vi "SelectMonitor.vi"(8 "Error In":errorcluster, 9 "Center?":bool, 10 "Monitor (0=primary)":u16, 11 "VI Path":path) -> (0 "Error out":errorcluster)   [LabVIEW 2012, in "LV-Utilities.lvlib"]
uses:
  LV-Utilities.lvlib
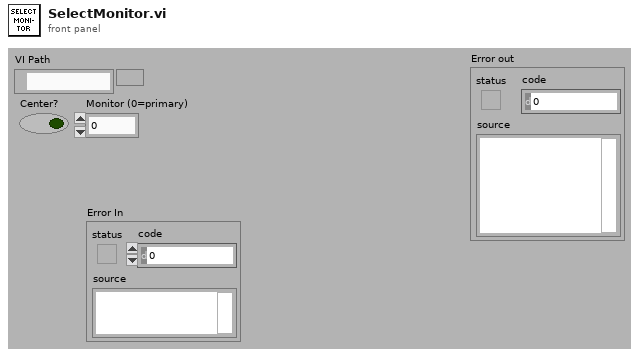
[diagram p1: front panel]
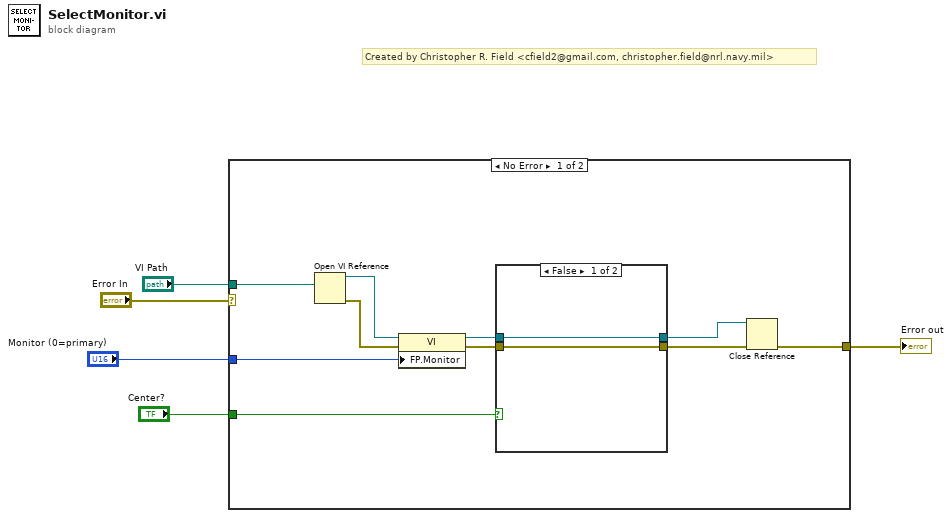
[diagram p0: block diagram]
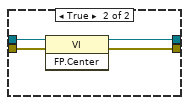
[diagram p2: hidden frame]
diagram:
  # "Created by Christopher R. Field <cfield2@gmail.com, christopher.field@nrl.navy.mil>"
  n1 = case shown="No Error" "Error In" {
    selector: "Error In" -> [_ w22]
    tunnel: [w13 w22] -> w5
    tunnel: "VI Path" -> [w12 _]
    tunnel: "Center?" -> [w7 _]
    tunnel: "Monitor (0=primary)" -> [w6 _]
    frame No Error {
      n2 = Open VI Reference(vi path=w12) -> (vi reference=w15:refnum<vi>, error out=w14:errorcluster)  [unwired: 5 in]
      n3 = property class="VI"(reference=w15, error in=w14, "FP.Monitor"=w6) -> (reference out=w11:refnum<vi>, error out=w10:errorcluster)
      n4 = case shown="False" w7 {
        tunnel: w11 -> [w17 w21]
        tunnel: w10 -> [w16 w20]
        tunnel: [w16 w19] -> w9
        tunnel: [w17 w18] -> w8
        frame False {
        }
        frame True {
          n5 = invoke class="VI" method="FP.Center"(reference=w21, error in=w20) -> (reference out=w18:refnum<vi>, error out=w19:errorcluster)  [unwired: 1 in, 1 out]
        }
      }
      n6 = Close Reference(reference=w8, error in (no error)=w9) -> (error out=w13:errorcluster)
    }
    frame Error {
    }
  }
  "Error out" <- w5
